vi "double_exponential_smoothing.vi"(2 "last_dema":dbl, 3 "last_ema":dbl, 4 "x":dbl, 5 "alpha":dbl) -> (0 "dema":dbl, 1 "ema":dbl)   [LabVIEW 2019]
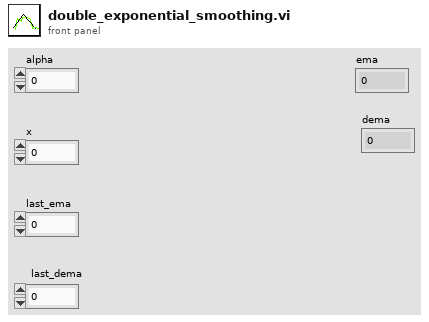
[diagram p1: front panel]
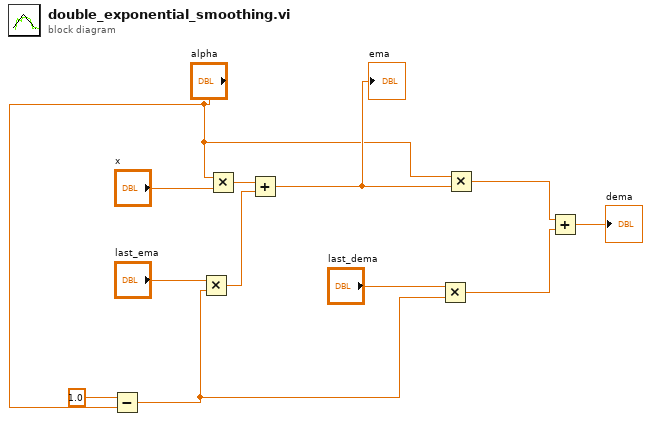
[diagram p0: block diagram]
diagram:
  n1 = Subtract(x=1.0, y="alpha") -> (x-y=w4:dbl)
  n2 = Multiply(x="last_ema", y=w4) -> (x*y=w8:dbl)
  n3 = Multiply(x="alpha", y="x") -> (x*y=w9:dbl)
  n4 = Add(x=w9, y=w8) -> (x+y=w7:dbl)
  "ema" <- w7
  n5 = Multiply(x="last_dema", y=w4) -> (x*y=w2:dbl)
  n6 = Multiply(x="alpha", y=w7) -> (x*y=w3:dbl)
  n7 = Add(x=w3, y=w2) -> (x+y=→"dema":dbl)
